vi "DSF.Engine.Execution.Builder.Set Status Pointers.vi"(8 "error in (no error)":errorcluster, 10 "Status Pointers":T1, 11 "Builder in":refnum<class "DSF.Engine.Execution.Builder.lvclass">) -> (0 "error out":errorcluster, 3 "Builder out":refnum<class "DSF.Engine.Execution.Builder.lvclass">)   [LabVIEW 2016, in "DSF.Engine.lvlib" / "DSF.Engine.Execution.Builder.lvclass"]
uses:
  Builder/DSF.Engine.Execution.Builder.lvclass
  DSF.Engine.Execution.Builder.Status Pointers.ctl
  Memory.Pointer/DSF.Memory.Pointer.U32.lvclass
  Builder/DSF.Engine.Execution.Builder.lvclass/DSF.Engine.Execution.Builder.ctl
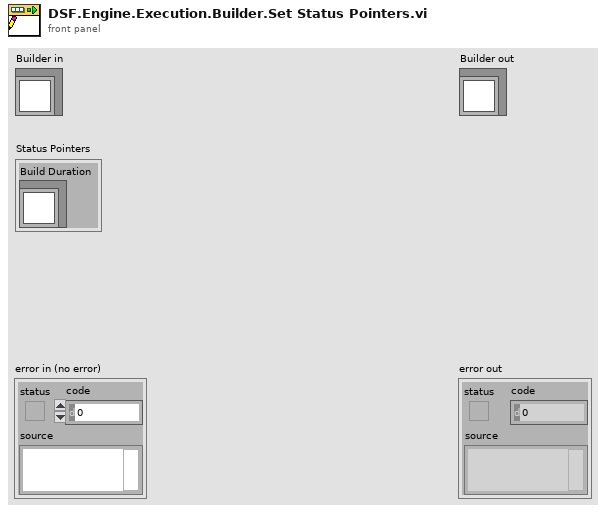
[diagram p1: front panel]
types:
  T1 = typedef "DSF.Engine.lvlib/DSF.Engine.Execution.Builder.lvclass/DSF.Engine.Execution.Builder.Status Pointers.ctl" = cluster{"Build Duration":refnum<class "DSF.Memory.Pointer.U32.lvclass">}
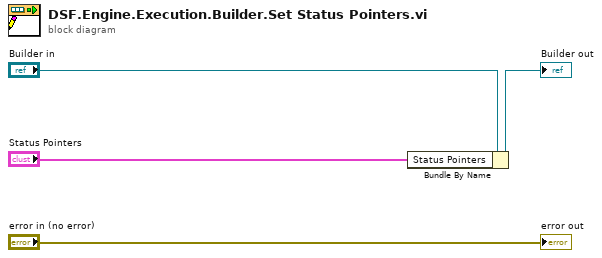
[diagram p0: block diagram]
diagram:
  n1 = Bundle By Name(cluster="Builder in", "Status Pointers"="Status Pointers") -> (→"Builder out":refnum<class "DSF.Engine.Execution.Builder.lvclass">)
  "error out" <- "error in (no error)"
